vi "Read N single images.vi"(6 "error in":errorcluster, 9 "Image info":T1(array[cluster])) -> (0 "error out":errorcluster, 1 "File paths out":path[](array[path]), 2 "Images out":T2[](array[typedef]), 3 "Image types out":u32[](array[numeric]))   [LabVIEW 2011]
doc: "Loads several different images, either from individual image files or from the specified frame of a tiff stack."
uses:
  <vilib>/vision/Image Controls.llb/IMAQ Image.ctl
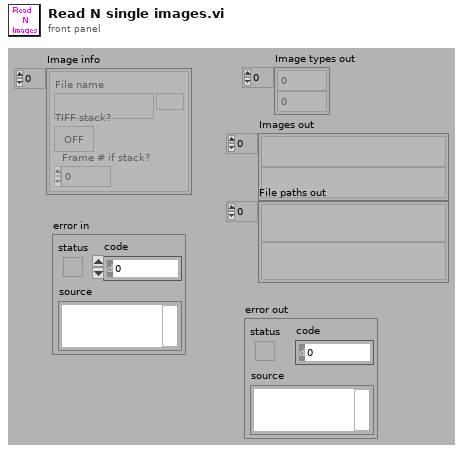
[diagram p1: front panel]
types:
  T1 = cluster{"File name":path, "TIFF stack?":bool, "Frame # if stack?":u32}[]
  T2 = typedef "IMAQ Image.ctl" = refnum<image>
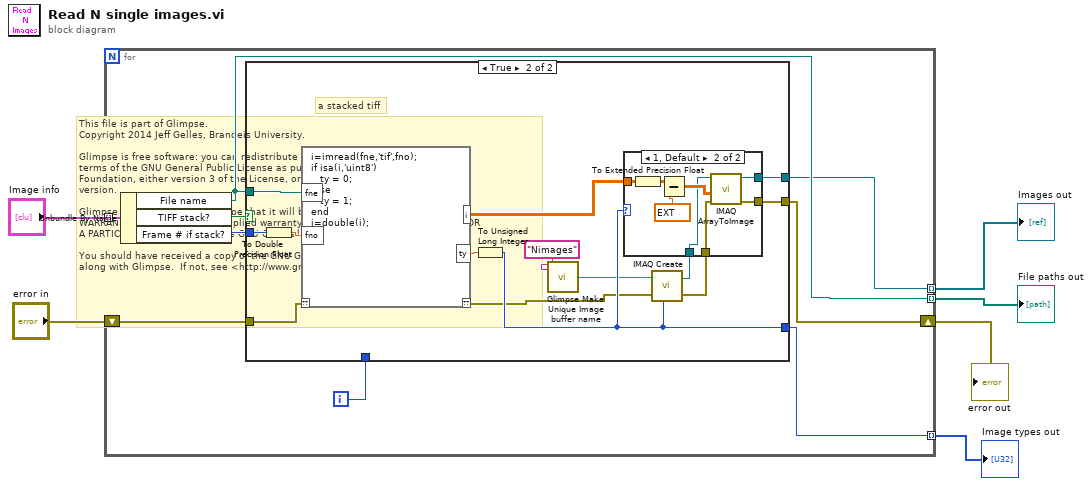
[diagram p0: block diagram]
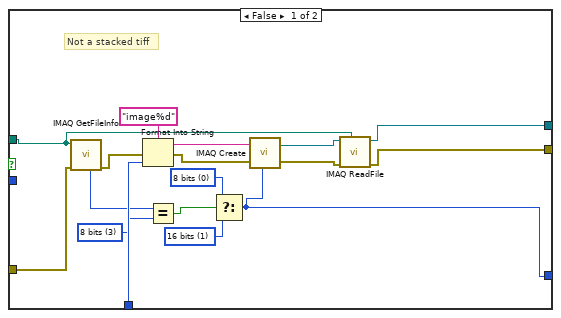
[diagram p2: hidden frame]
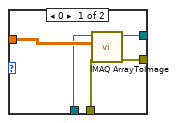
[diagram p3: hidden frame]
diagram:
  # "This file is part of Glimpse. \nCopyright 2014 Jeff Gelles, Brandeis University.    \n\nGlimpse is free software: you can redistribute it and/or modify it under the \nterms of the GNU General Public License as published by the Free Software \nFoundation, either version 3 of the License, or (at your option) any later \nversion.\n\nGlimpse is distributed in the hope that it will be useful, but WITHOUT ANY \nWARRANTY; without even the implied warranty of MERCHANTABILITY or FITNESS FOR \nA PARTICULAR PURPOSE.  See the GNU General Public License for more details.\n\nYou should have received a copy of the GNU General Public License\nalong with Glimpse.  If not, see <http://www.gnu.org/licenses/>."
  n1 = for {
    tunnel: "Image info" -> [w15] mode=indexing
    shift-right: [w8] -> w4
    shift-left: "error in" -> [w12]
    tunnel: [w10] -> w5 mode=indexing
    tunnel: [w9] -> w6 mode=indexing
    tunnel: [w7] -> w1 mode=indexing
    i -> [w11]
    n2 = Unbundle By Name(w15) -> ("File name"=w10:path, "TIFF stack?"=w14:bool, "Frame # if stack?"=w13:u32)
    n3 = case shown="True" w14 {
      tunnel: w10 -> [w18 w46]
      tunnel: w13 -> [_ w45]
      tunnel: [w21 w40] -> w7
      tunnel: w12 -> [w30 w43]
      tunnel: w11 -> [w28 _]
      tunnel: [w16 w38] -> w9
      tunnel: [w17 w37] -> w8
      frame False {
        w24 = 3 items=["1 bit", "2 bits", "4 bits", "8 bits", "12 bits (unsigned)", "16 bits (unsigned)", "16 bits (signed)", "16 bits (RGB chunky)", "24 bits (RGB chunky)", "24 bits (RGB planar)", "32 bits (unsigned)", "32 bits (signed)", "32 bits (RGB chunky)", "32 bits (float)", "48 bits (Complex 2x24 int)", "64 bits (Complex 2x32 float)", "reserved", "24 bits (HSL)"] ("File Data Type")
        w26 = u32 1 items=["8 bits", "16 bits", "Float", "Complex", "RGB", "HSL"] ("Image Type")
        w25 = u32 0 items=["8 bits", "16 bits", "Float", "Complex", "RGB", "HSL"] ("Image Type")
        # "Not a stacked tiff"
        n4 = call "IMAQ GetFileInfo"("error in (no error)"=w30, "File Path"=w18) -> ("error out"=w27:errorcluster, "File Data Type"=w23:i32)  [unwired: 8 out]
        n5 = Format Into String(format string="image%d", error in=w27, w28) -> (resulting string=w31:string, error out=w32:errorcluster)  [unwired: 1 in]
        n6 = Equal?(x=w23, y=w24) -> (x = y?=w22:bool)
        n7 = Select(t=w25, s=w22, f=w26) -> (s? t:f=w21:u32)
        n8 = call "IMAQ Create"("Image Name"=w31, "Image Type"=w21, "error in (no error)"=w32) -> ("New Image"=w19:T2, "error out"=w20:errorcluster)  [unwired: 1 in, 1 out]
        n9 = call "IMAQ ReadFile"("File Path"=w18, "error in (no error)"=w20, "Image"=w19) -> ("error out"=w17:errorcluster, "Image Out"=w16:T2)  [unwired: 2 in, 5 out]
      }
      frame True {
        # "a stacked tiff"
        n10 = To Double Precision Float(number=w45) -> (double precision float=w36:dbl)
        n11 = script code="i=imread(fne,'tif',fno);\nif isa(i,'uint8')\n   ty = 0;\nelse\n   ty = 1;\nend\ni=double(i);"("??"=w43, "fne"=w46, "fno"=w36) -> ("??"=w33:errorcluster, "i"=w41:dbl[][], "ty"=w44:dbl)
        n12 = To Unsigned Long Integer(number=w44) -> (unsigned 32bit integer=w40:u32)
        n13 = call "Glimpse Make Unique Image buffer name.vi"("Buffer  base name"="Nimages" ("format string")) -> ("Image Name"=w35:string)  [unwired: 1 out]
        n14 = call "IMAQ Create"("Image Name"=w35, "Image Type"=w40, "error in (no error)"=w33) -> ("New Image"=w39:T2, "error out"=w42:errorcluster)  [unwired: 1 in, 1 out]
        n15 = case shown="1, Default" w40 {
          tunnel: [w51 w57] -> w38
          tunnel: w42 -> [w49 w56]
          tunnel: w41 -> [w48 w55]
          tunnel: w39 -> [w47 w54]
          tunnel: [w50 w53] -> w37
          frame 0 {
            n16 = call "IMAQ ArrayToImage"("error in (no error)"=w49, "Image Pixels (U8)"=w48, "Image"=w47) -> ("error out"=w50:errorcluster, "Image Out"=w51:T2)  [unwired: 3 in, 4 out]
          }
          frame 1, Default {
            n17 = To Extended Precision Float(1:w55) -> (0:w52:ext[][])
            n18 = Subtract(x=w52, y=ext 32767.0) -> (x-y=w58:ext[][])
            n19 = call "IMAQ ArrayToImage"("error in (no error)"=w56, "Image Pixels (I16)"=w58, "Image"=w54) -> ("error out"=w53:errorcluster, "Image Out"=w57:T2)  [unwired: 3 in, 4 out]
          }
        }
      }
    }
  }
  "Images out" <- w6
  "File paths out" <- w5
  "error out" <- w4
  "Image types out" <- w1
